vi "WPI_AnalogOutputOpen.vi"(8 "error in (no error)":errorcluster, 10 "AO Channel":T1) -> (0 "error out":errorcluster, 3 "AODeviceRef":T2)   [LabVIEW 2017]
doc: "Opens a reference to the analog output channel you specify. You must open a reference before using any other Analog Output VIs.\n\nThis software is licensed. Open the labview\\readme\\WPI Robotics Library Open Source License.txt file for more information."
uses:
  <vilib>/Rock Robotics/WPI/AnalogOutput/WPI_AOChannelDevRef.ctl
  <vilib>/Rock Robotics/WPI/AnalogOutput/WPI_AnalogOutputChannel.ctl
  <vilib>/Rock Robotics/WPI/AnalogChannel/WPI_AnalogChannelChannelCacheOp.ctl
  <vilib>/Rock Robotics/SystemInterfaces/NetworkCommunication/NetComm_UsageReport_ResourceType.ctl
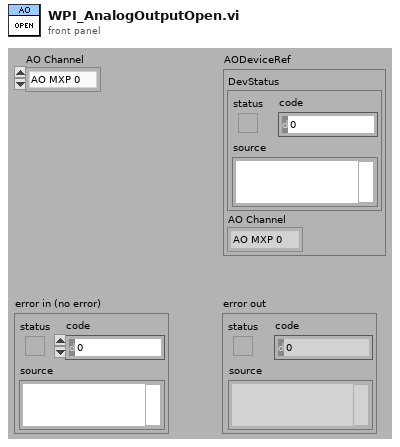
[diagram p1: front panel]
types:
  T1 = typedef "WPI_AnalogOutputChannel.ctl" = enum8{"AO MXP 0", "AO MXP 1", "Invalid"}
  T2 = typedef "WPI_AOChannelDevRef.ctl" = cluster{"DevStatus":errorcluster, "AO Channel":T1}
  T3 = typedef "FPGA_SystemFRC FPGA Ref.ctl" = refnum<k20>
  T4 = typedef "NetComm_UsageReport_ResourceType.ctl" = enum8{"Controller", "Module", "Language", "CANPlugin", "Accelerometer", "ADXL345", "AnalogChannel", "AnalogTrigger", "AnalogTriggerOutput", "CANJaguar", "Compressor", "Counter", "Dashboard", "DigitalInput", "DigitalOutput", "DriverStationCIO", "DriverStationEIO", "DriverStationLCD", "Encoder", "GearTooth", "Gyro", "I2C", "Framework", "Jaguar", "Joystick", "Kinect", "KinectStick", "PIDController", "Preferences", "PWM", "Relay", "RobotDrive", "SerialPort", "Servo", "Solenoid", "SPI", "Task", "Ultrasonic", "Victor", "Button", "Command", "AxisCamera", "PCVideoServer", "SmartDashboard", "Talon", "HiTechnicColorSensor", "HiTechnicAccel", "HiTechnicCompass", "SRF08", "AnalogOutput", "Victor SP", "Talon SRX", "CAN Talon SRX", "ADXL362 Accel", "ADXRS450 Gyro", "Rev SPARK", "Mindsensors SD540", "Digital Filter", "ADIS16448", "PDP", "PCM", "PigeonIMU", "Nidec Brushless", "CTRE CANifier", "CTRE Future 0", "CTRE Future 1", "CTRE Future 2", "CTRE Future 3", "CTRE Future 4", "CTRE Future 5", "CTRE Future 6"}
  T5 = typedef "WPI_AnalogChannelChannelCacheOp.ctl" = enum16{"Acquire", "Release", "Status"}
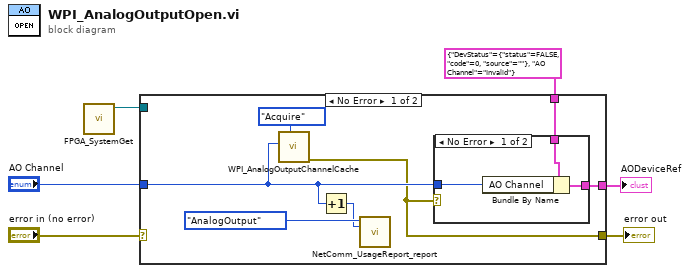
[diagram p0: block diagram]
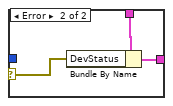
[diagram p2: hidden frame]
diagram:
  n1 = call <vilib>:"FPGA_SystemGet.vi"() -> ("FRC FPGA Ref"=w1:T3)  [unwired: 2 in, 9 out]
  n2 = case shown="No Error" "error in (no error)" {
    selector: "error in (no error)" -> [_ w20]
    tunnel: T2 {"DevStatus"={"status"=FALSE, "code"=0, "source"=""}, "AO Channel"=enum."Invalid"} ("AODeviceRef") -> [w13 w21]
    tunnel: [w12 w21] -> w3
    tunnel: "AO Channel" -> [w9 _]
    tunnel: [w7 w20] -> w4
    tunnel: w1 -> [_ _]
    frame No Error {
      n3 = call <vilib>:"WPI_AnalogOutputChannelCache.vi"("Operation"=WPI_AnalogChannelChannelCacheOp."Acquire", "AO Channel"=w9) -> ("error out"=w7:errorcluster)  [unwired: 7 in, 2 out]
      n4 = Increment(x=w9) -> (x+1=w8:T1)
      n5 = call <vilib>:"NetComm_UsageReport_report.vi"("Instance Number"=w8, "Resource Type"=NetComm_UsageReport_ResourceType."AnalogOutput") -> ()  [unwired: 10 in]
      n6 = case shown="No Error" w7 {
        selector: w7 -> [_ w17]
        tunnel: w13 -> [w16 w19]
        tunnel: [w15 w18] -> w12
        tunnel: w9 -> [w14 _]
        frame No Error {
          n7 = Bundle By Name(cluster=w16, "AO Channel"=w14) -> (w15:T2)
        }
        frame Error {
          n8 = Bundle By Name(cluster=w19, "DevStatus"=w17) -> (w18:T2)
        }
      }
    }
    frame Error {
    }
  }
  "AODeviceRef" <- w3
  "error out" <- w4
